vi "Cleanup Engine Stream.vi"(8 "error in (no error)":errorcluster, 11 "Refs":T1) -> (0 "error out":errorcluster)   [LabVIEW 2019, in "CAN Streaming Support Engine.lvlib"]
uses:
  CAN Streaming Support Engine.lvlib
  Types/Engine Stream API Refs.ctl
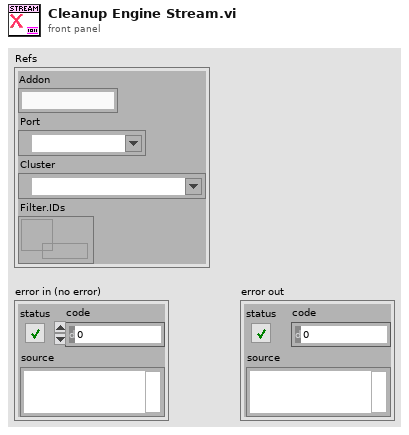
[diagram p1: front panel]
types:
  T1 = typedef "CAN Streaming Support Engine.lvlib/Engine Stream API Refs.ctl" = cluster{"Addon":string, "Port":refnum<k21>, "Cluster":refnum<k21>, "Filter.IDs":refnum<data-value>}
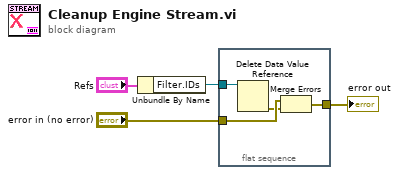
[diagram p0: block diagram]
diagram:
  n1 = Unbundle By Name("Refs") -> ("Filter.IDs"=w4:refnum<data-value>)
  n2 = flat-sequence {
    tunnel: "error in (no error)" -> [w8]
    tunnel: [w6] -> w2
    tunnel: w4 -> [w5]
    frame #0 {
      n3 = Delete Data Value Reference(data value reference=w5) -> (error out=w7:errorcluster)  [unwired: 1 in, 1 out]
      n4 = Merge Errors(w8, w7) -> (w6:errorcluster)
    }
  }
  "error out" <- w2
